vi "StandAlone_ReadData.vi"() -> ()   [LabVIEW 2019]
uses:
  Controls/PlotColorArray.ctl
  <vilib>/Utility/file.llb/Read Delimited Spreadsheet (string).vi
panel:
  in  "Finish This Run's Data Processing":bool
  in  "Adjust Axis":bool
  in  "Minimum Current (V)":dbl
  in  "Maximum Voltage (V)":dbl
  in  "Time Maximum":dbl
  in  "Time Minimum":dbl
  in  "Maximum Current (A)":dbl
  in  "Minimum Current (A)":dbl
  in  "Decimal Place":string="8"
  in  "Copied Directory":path=path "C:/testnull"
  out "Channel Begin Processed":string
  out "all rows":string[][](array[string])
  out "Current Measurements":cluster{dbl[], dbl[]}[](graph)
  out "Voltage Measurements":cluster{dbl[], dbl[]}[](graph)
  in  "Run Number":string
  # "Please review the legend. The plot names/colors may have switched from the collection phase"
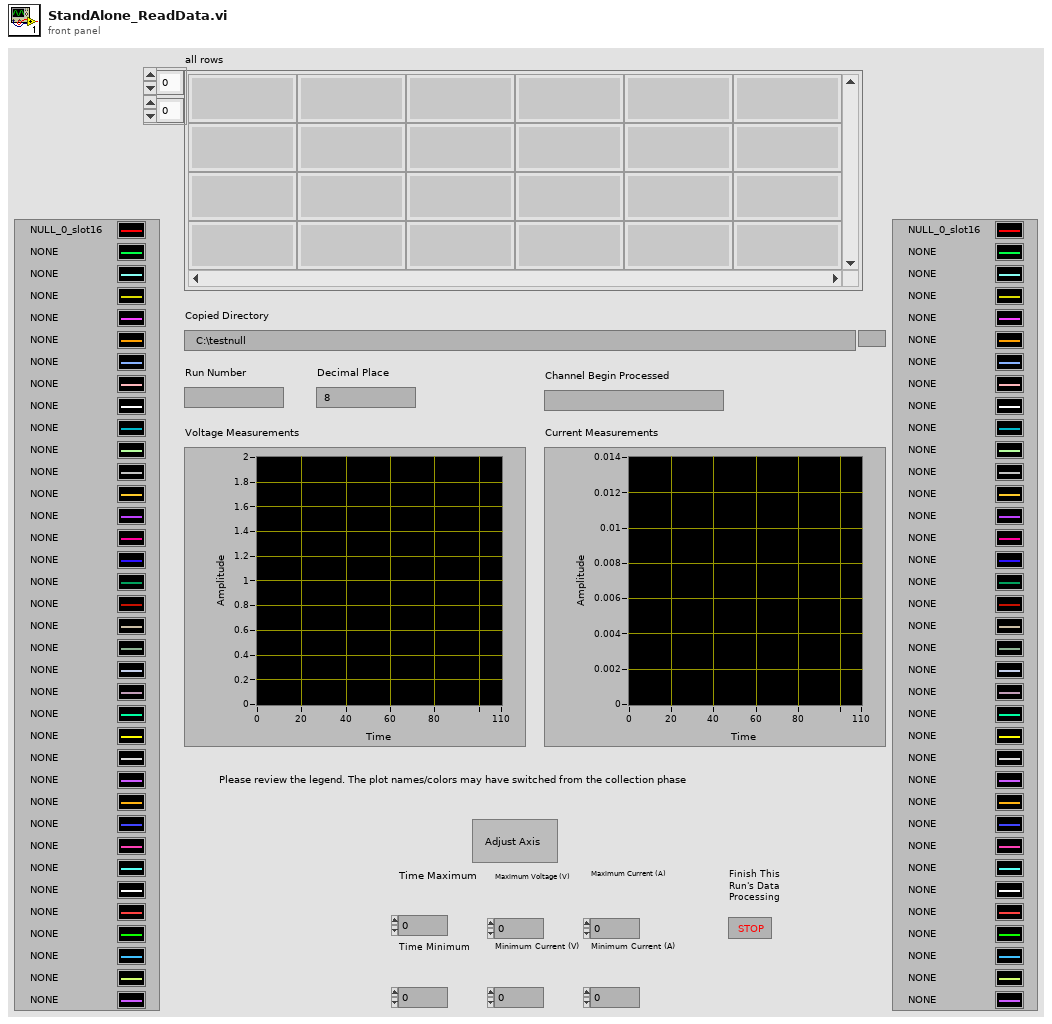
[diagram p1: front panel]
types:
  T1 = typedef "PlotColorArray.ctl" = u32[]
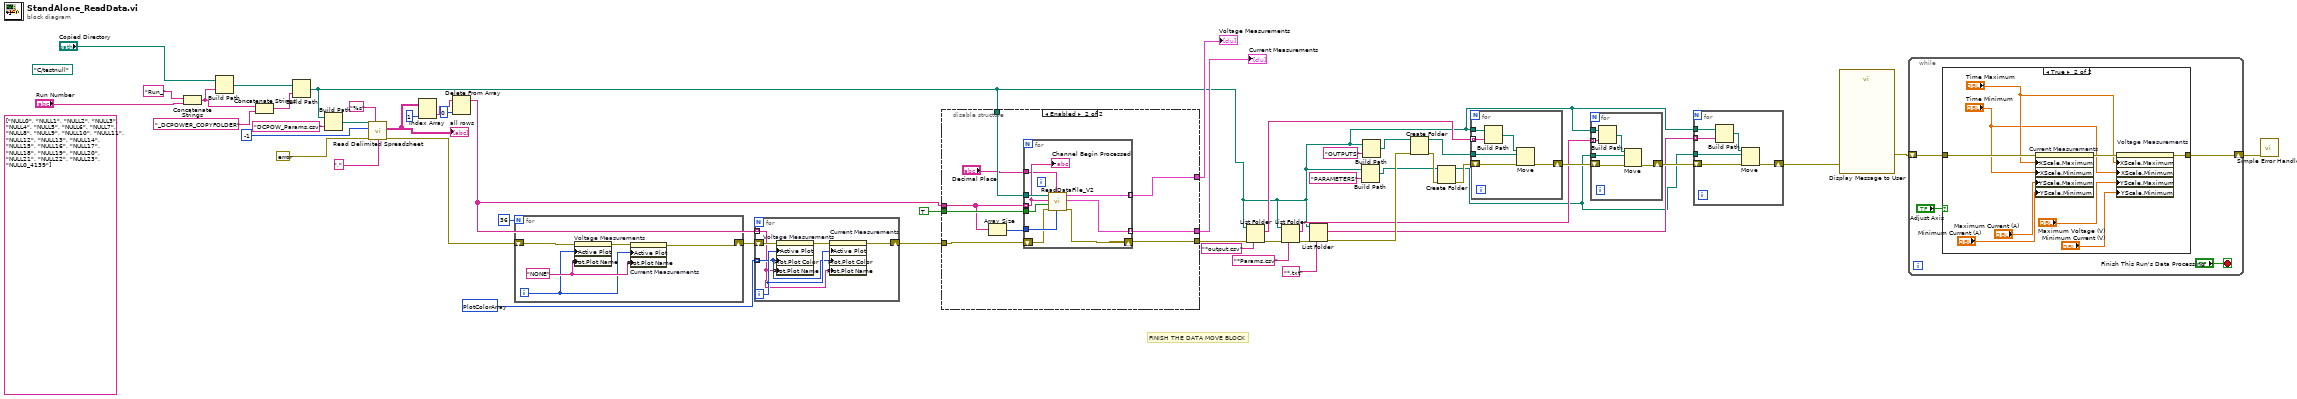
[diagram p0: block diagram]
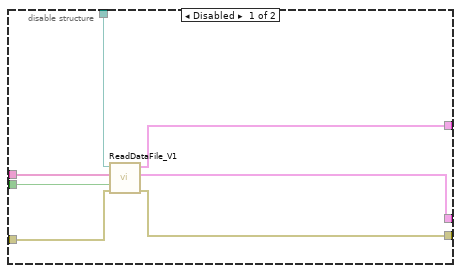
[diagram p3: hidden frame]
diagram:
  (unwired) path "C:/testnull" ("base path")
  (unwired) string[] ["NULL0", "NULL1", "NULL2", "NULL3", "NULL4", "NULL5", "NULL6", "NULL7", "NULL8", "NULL9", "NULL10", "NULL11", "NULL12", "NULL13", "NULL14", "NULL15", "NULL16", "NULL17", "NULL18", "NULL19", "NULL20", "NULL21", "NULL22", "NULL23", "NULL0_4139"]
  # "FINISH THE DATA MOVE BLOCK"
  n1 = Concatenate Strings("Run_" ("string"), "Run Number") -> (w45:string)
  n2 = Build Path(base path="Copied Directory", name or relative path=w45) -> (appended path=w48:path)
  n3 = Concatenate Strings(w45, "_DCPOWER_COPYFOLDER" ("string")) -> (w47:string)
  n4 = Build Path(base path=w48, name or relative path=w47) -> (appended path=w6:path)
  n5 = Build Path(base path=w6, name or relative path="DCPOW_Params.csv") -> (appended path=w43:path)
  n6 = call-poly <vilib>:"Read Delimited Spreadsheet.vi"("file path (dialog if empty)"=w43, "format (%s)"="%s" ("format (%.3f)"), "number of rows (all:-1)"=-1, "error in (no error)"=errorcluster {"status"=FALSE, "code"=0, "source"=""}, "delimiter (\\t)"="," ("delimiter (\\t)")) -> ("all rows"=w38:string[][], "error out"=w33:errorcluster)  [unwired: 5 in, 4 out]
  "all rows" <- w38
  n7 = Index Array(array=w38, index (col)=1 ("disabled index (col)")) -> (element=w36:string[])  [unwired: 1 in]
  n8 = Delete From Array(array=w36, index=0) -> (array with subset deleted=w27:string[])  [unwired: 1 in, 1 out]
  n9 = for {
    N: 36 -> [_]
    shift-right: [w53] -> w32
    shift-left: w33 -> [w55]
    i -> [w51]
    w52 = "NONE" ("Plot.Plot Name")
    n10 = property on="Voltage Measurements" class="XYGraph (strict)"(error in=w55, "Active Plot"=w51, "Plot.Plot Name"=w52) -> (error out=w54:errorcluster)  [unwired: 1 in, 1 out]
    n11 = property on="Current Measurements" class="XYGraph (strict)"(error in=w54, "Active Plot"=w51, "Plot.Plot Name"=w52) -> (error out=w53:errorcluster)  [unwired: 1 in, 1 out]
  }
  n12 = for {
    shift-right: [w59] -> w34
    shift-left: w32 -> [w61]
    tunnel: w27 -> [w56] mode=indexing
    tunnel: T1 [16711686, 65351, 8978420, 14474240, 16139007, 16752640, 8958719, 16758973, 16777215, 46792, 11992992, 12961221, 16763690, 12600063, 16711835, 2953983, 40796, 13111296, 13352613, 9221011, 12964076, 12819897, 65442, 16776704, 14540253, 16740729, 10658047, 10813344, 16753521, 13413843, 8691115, 10339240, 14401205, 16746704, 7467519, 16775978, 13872558, 11387603, 13354405, 10420227, 13107364, 4060, 35208, 11817216, 7566080, 40796, 7539456, 2837073, 6372186, 7499083, 10648702, 16757152] ("Array") -> [w57] mode=indexing
    i -> [w58]
    n13 = property on="Voltage Measurements" class="XYGraph (strict)"(error in=w61, "Active Plot"=w58, "Plot.Plot Color"=w57, "Plot.Plot Name"=w56) -> (error out=w60:errorcluster)  [unwired: 1 in, 1 out]
    n14 = property on="Current Measurements" class="XYGraph (strict)"(error in=w60, "Active Plot"=w58, "Plot.Plot Color"=w57, "Plot.Plot Name"=w56) -> (error out=w59:errorcluster)  [unwired: 1 in, 1 out]
  }
  n15 = disable-structure shown="Enabled" {
    disable-tunnel: w27 -> [w68 w74]
    disable-tunnel: w6 -> [w67 w77]
    disable-tunnel: w34 -> [w66 w71]
    disable-tunnel: [w65 w70] -> w24
    disable-tunnel: [w64 w72] -> w30
    disable-tunnel: [w63 w73] -> w29
    disable-tunnel: TRUE ("Create CSV files?") -> [w62 w76]
    frame Disabled {
      n16 = call "ReadDataFile_V1.vi"("error in (no error)"=w66, "Create CSV files?"=w62, "Channel Names Array"=w68, "DataFolder Path"=w67) -> ("error out"=w65:errorcluster, "Current Measurements"=w64:cluster{dbl[], dbl[]}[], "Voltage Measurements"=w63:cluster{dbl[], dbl[]}[])  [unwired: 5 in]
    }
    frame Enabled {
      n17 = Array Size(array=w74) -> (size(s)=w75:i32)
      n18 = for {
        tunnel: w77 -> [w86]
        tunnel: w74 -> [w85] mode=indexing
        tunnel: w76 -> [w84]
        tunnel: w75 -> [w83]
        tunnel: [w82] -> w73 mode=indexing
        tunnel: [w81] -> w72 mode=indexing
        shift-right: [w79] -> w70
        shift-left: w71 -> [w80]
        tunnel: "Decimal Place" -> [w78]
        n19 = call "ReadDataFile_V2.vi"("Channel Name Array Size"=w83, "Resolution"=w78, "error in (no error)"=w80, "Create CSV files?"=w84, "Channel Name Individual"=w85, "DataFolder Path"=w86) -> ("error out"=w79:errorcluster, "Current Measurements Individual"=w81:cluster{dbl[], dbl[]}, "Voltage Measurements Individual"=w82:cluster{dbl[], dbl[]})  [unwired: 3 in]
        "Channel Begin Processed" <- w85
      }
    }
  }
  "Voltage Measurements" <- w29
  "Current Measurements" <- w30
  n20 = List Folder(path=w6, pattern="*output.csv", error in=w24) -> (filenames=w12:string[], error out=w22:errorcluster)  [unwired: 1 in, 2 out]
  n21 = List Folder(path=w6, pattern="*Params.csv", error in=w22) -> (filenames=w8:string[], error out=w20:errorcluster)  [unwired: 1 in, 2 out]
  n22 = List Folder(path=w6, pattern="*.txt", error in=w20) -> (filenames=w5:string[], error out=w16:errorcluster)  [unwired: 1 in, 2 out]
  n23 = Build Path(base path=w6, name or relative path="PARAMETERS") -> (appended path=w14:path)
  n24 = Build Path(base path=w6, name or relative path="OUTPUTS") -> (appended path=w13:path)
  n25 = Create Folder(path (use dialog)=w13, error in=w16) -> (created path=w9:path, error out=w15:errorcluster)  [unwired: 1 in, 1 out]
  n26 = Create Folder(path (use dialog)=w14, error in=w15) -> (created path=w4:path, error out=w10:errorcluster)  [unwired: 1 in, 1 out]
  n27 = for {
    tunnel: w6 -> [w92]
    tunnel: w12 -> [w91] mode=indexing
    shift-right: [w90] -> w11
    shift-left: w10 -> [w89]
    tunnel: w9 -> [w87]
    n28 = Build Path(base path=w92, name or relative path=w91) -> (appended path=w88:path)
    n29 = Move(source path=w88, error in=w89, 10:w87) -> (error out=w90:errorcluster)  [unwired: 2 in, 2 out]
  }
  n30 = for {
    tunnel: w6 -> [w96]
    shift-right: [w97] -> w7
    shift-left: w11 -> [w98]
    tunnel: w8 -> [w95] mode=indexing
    tunnel: w4 -> [w93]
    n31 = Build Path(base path=w96, name or relative path=w95) -> (appended path=w94:path)
    n32 = Move(source path=w94, error in=w98, 10:w93) -> (error out=w97:errorcluster)  [unwired: 2 in, 2 out]
  }
  n33 = for {
    shift-right: [w102] -> w3
    shift-left: w7 -> [w103]
    tunnel: w6 -> [w101]
    tunnel: w5 -> [w100] mode=indexing
    tunnel: w4 -> [w99]
    n34 = Build Path(base path=w101, name or relative path=w100) -> (appended path=w104:path)
    n35 = Move(source path=w104, error in=w103, 10:w99) -> (error out=w102:errorcluster)  [unwired: 2 in, 2 out]
  }
  n36 = call "Display Message to User"("error in (no error)"=w3) -> ("error out"=w2:errorcluster)  [unwired: 9 in, 1 out]
  n37 = while {
    shift-right: [w107] -> w1
    shift-left: w2 -> [w108]
    stop <- "Finish This Run's Data Processing" stop-if-true
    n38 = case shown="True" "Adjust Axis" {
      tunnel: w108 -> [w109 w118]
      tunnel: [w109 w116] -> w107
      frame False {
      }
      frame True {
        n39 = property on="Current Measurements" class="XYGraph (strict)"(error in=w118, "XScale.Maximum"="Time Maximum", "XScale.Minimum"="Time Minimum", "YScale.Maximum"="Maximum Current (A)", "YScale.Minimum"="Minimum Current (A)") -> (error out=w117:errorcluster)  [unwired: 1 in, 1 out]
        n40 = property on="Voltage Measurements" class="XYGraph (strict)"(error in=w117, "XScale.Maximum"="Time Maximum", "XScale.Minimum"="Time Minimum", "YScale.Maximum"="Maximum Voltage (V)", "YScale.Minimum"="Minimum Current (V)") -> (error out=w116:errorcluster)  [unwired: 1 in, 1 out]
      }
    }
  }
  n41 = call <vilib>:"Simple Error Handler.vi"("error in (no error)"=w1) -> ()  [unwired: 4 in, 5 out]
